vi "scp_recv.vi"() -> ()   [LabVIEW 2013]
doc: "Illustrates how to receive a file from a remote server via SCP."
uses:
  libssh2/libssh2_init_default.vi
  libssh2/libssh2_session_handshake_tcp.vi
  libssh2/libssh2.lvlib
panel:
  out "content":string
  out "size":i64
  out "mode":u16 format="%.0o"
  out "access time":timestamp
  out "modified time":timestamp
  out "error message":string
  in  "file":string="/"
  out "error out":errorcluster
  in  "password":string
  in  "username":string
  in  "hostname":string
  # "Remote file information"
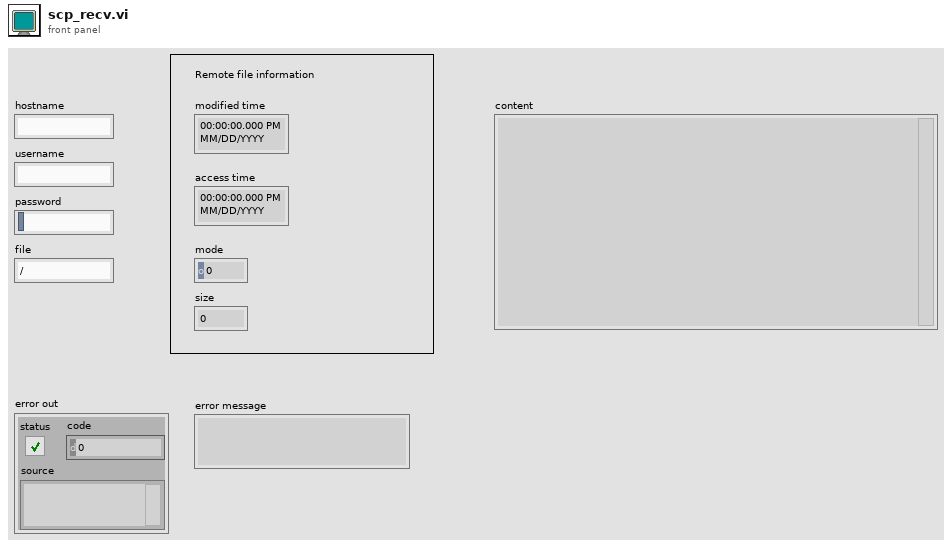
[diagram p1: front panel]
types:
  T1 = typedef "libssh2.lvlib/Session Refnum.ctl" = refnum<k1>
  T2 = typedef "libssh2.lvlib/libssh2_struct_stat.ctl" = cluster{"st_dev":u64, "st_ino":u16, "st_mode":u16, "st_nlink":i16, "st_uid":i16, "st_gid":i16, "st_rdev":u32, "st_size":i64, "st_atime":i64, "st_mtime":i64, "st_ctime":i64}
  T3 = typedef "libssh2.lvlib/Channel Refnum.ctl" = refnum<k1>
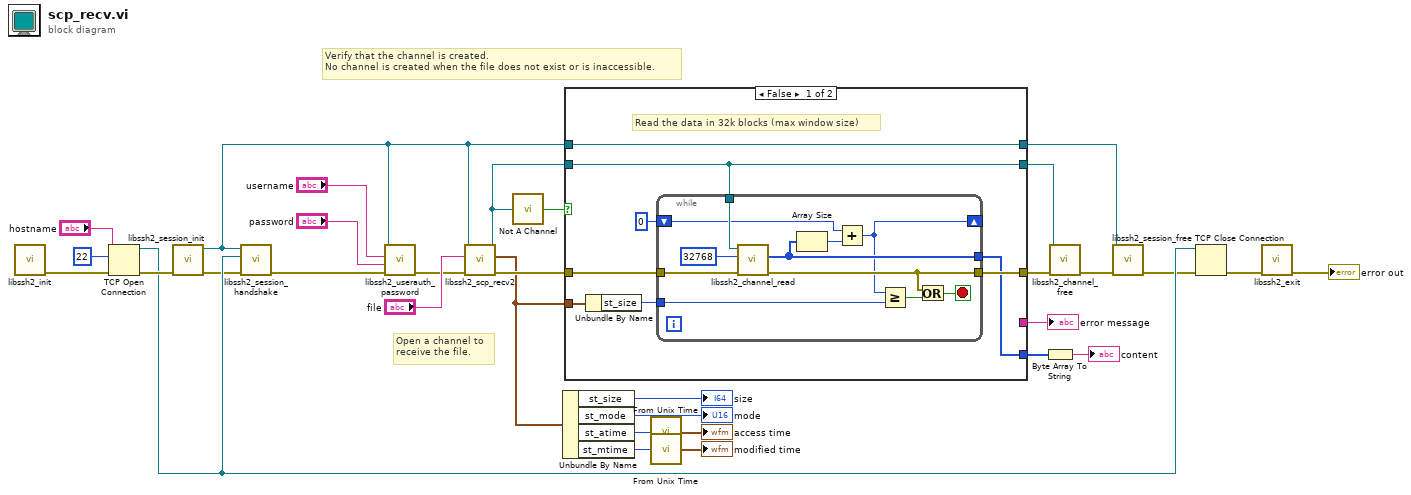
[diagram p0: block diagram]
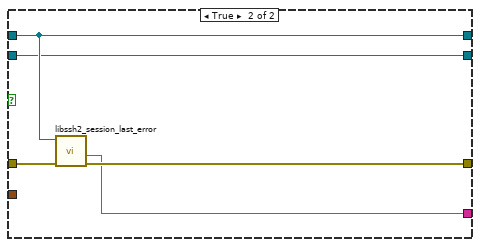
[diagram p2: hidden frame]
diagram:
  # "Verify that the channel is created.\nNo channel is created when the file does not exist or is inaccessible."
  # "Open a channel to\nreceive the file."
  n1 = call-poly "libssh2_init.vi"() -> ("error out"=w31:errorcluster)  [unwired: 11 in]
  n2 = TCP Open Connection(address="hostname", remote port or service name=u16 22, error in (no error)=w31) -> (connection ID=w29:refnum<k5>, error out=w30:errorcluster)  [unwired: 2 in]
  n3 = call "libssh2_session_init.vi"("error in (no error)"=w30) -> ("error out"=w28:errorcluster, "session"=w16:T1)  [unwired: 9 in]
  n4 = call-poly "libssh2_session_handshake.vi"("error in (no error)"=w28, "tcp connection"=w29, "session"=w16) -> ("error out"=w32:errorcluster)  [unwired: 8 in]
  n5 = call "libssh2_userauth_password.vi"("error in (no error)"=w32, "password"="password", "username"="username", "session"=w16) -> ("error out"=w19:errorcluster)  [unwired: 7 in]
  n6 = call "libssh2_scp_recv2.vi"("error in (no error)"=w19, "path"="file", "session"=w16) -> ("error out"=w18:errorcluster, "stat"=w1:T2, "channel"=w13:T3)  [unwired: 6 in]
  n7 = call "Not A Channel.vi"("channel"=w13) -> ("Not a Channel?"=w17:bool)
  n8 = Unbundle By Name(w1) -> ("st_size"=→"size":i64, "st_mode"=→"mode":u16, "st_atime"=w7:i64, "st_mtime"=w8:i64)
  n9 = case shown="False" w17 {
    tunnel: w18 -> [w39 w56]
    tunnel: w16 -> [w40 w55]
    tunnel: [w40 w55] -> w15
    tunnel: [w38 w54] -> w10
    tunnel: [_ w53] -> w14
    tunnel: w13 -> [w37 w52]
    tunnel: [w37 w52] -> w12
    tunnel: [w33 _] -> w3
    tunnel: w1 -> [w34 _]
    frame False {
      # "Read the data in 32k blocks (max window size)"
      n10 = Unbundle By Name(w34) -> ("st_size"=w35:i64)
      n11 = while {
        tunnel: w39 -> [w51]
        tunnel: [w48] -> w38
        tunnel: w37 -> [w50]
        tunnel: [w45] -> w33 mode=concatenating
        tunnel: [w45] -> _
        shift-right: [w42] -> _
        shift-left: 0 -> [w43]
        tunnel: w35 -> [w41]
        stop <- w46 stop-if-true
        n12 = call "libssh2_channel_read.vi"("error in (no error)"=w51, "buffer length"=32768, "channel"=w50) -> ("error out"=w48:errorcluster, "buffer"=w45:u8[])  [unwired: 7 in]
        n13 = Array Size(array=w45) -> (size(s)=w44:i32)
        n14 = Add(x=w43, y=w44) -> (x+y=w42:i32)
        n15 = Greater Or Equal?(x=w42, y=w41) -> (x >= y?=w47:bool)
        n16 = Or(x=w48, y=w47) -> (x .or. y?=w46:bool)
      }
    }
    frame True {
      n17 = call "libssh2_session_last_error.vi"("error in (no error)"=w56, "session"=w55) -> ("error out"=w54:errorcluster, "error message"=w53:string)  [unwired: 7 in, 1 out]
    }
  }
  "error message" <- w14
  n18 = call "From Unix Time.vi"("unix time"=w7) -> ("timestamp"=→"access time":timestamp)  [unwired: 1 in]
  n19 = call "From Unix Time.vi"("unix time"=w8) -> ("timestamp"=→"modified time":timestamp)  [unwired: 1 in]
  n20 = Byte Array To String(unsigned byte array=w3) -> (string=→"content":string)
  n21 = call "libssh2_channel_free.vi"("error in (no error)"=w10, "channel"=w12) -> ("error out"=w11:errorcluster)  [unwired: 9 in]
  n22 = call "libssh2_session_free.vi"("error in (no error)"=w11, "session"=w15) -> ("error out"=w22:errorcluster)  [unwired: 9 in]
  n23 = TCP Close Connection(connection ID=w29, error in (no error)=w22) -> (error out=w21:errorcluster)  [unwired: 1 in, 1 out]
  n24 = call "libssh2_exit.vi"("error in (no error)"=w21) -> ("error out"=→"error out":errorcluster)  [unwired: 10 in]
